vi "FPGA_CounterReadTimerOutput.vi"(8 "error in (no error)":errorcluster, 11 "Ctr Ref in":T1={"DevStatus"={"status"=FALSE, "code"=0, "source"=""}, "CntIndex"=enum."Ctr 1"}) -> (0 "error out":errorcluster, 1 "Stalled":bool, 2 "Period (s)":dbl, 3 "Ctr Ref out":T1={"DevStatus"={"status"=FALSE, "code"=0, "source"=""}, "CntIndex"=enum."Ctr 1"})   [LabVIEW 2017]
uses:
  <vilib>/Rock Robotics/SystemInterfaces/Counter/FPGA_CounterCtrDevRef.ctl
  <vilib>/Rock Robotics/SystemInterfaces/Counter/FPGA_CounterCtrSystemIndex.ctl
  <vilib>/Rock Robotics/SystemInterfaces/System/FPGA_SystemFPGA Ref Global.vi
  <vilib>/Utility/error.llb/Error Cluster From Error Code.vi
  <vilib>/rvi/errors/niLvFpgaAdjustHostInterfaceError.vi
  <vilib>/rvi/interface/nirviReadWriteControl/nirviReadWriteControl.xnode
  <vilib>/Rock Robotics/SystemInterfaces/System/FPGA_SystemFRC FPGA Ref.ctl
  NiFpgaLv.dll
  <vilib>/rvi/interface/Simulation/niFpgaSimulationCallBeginRW.vi
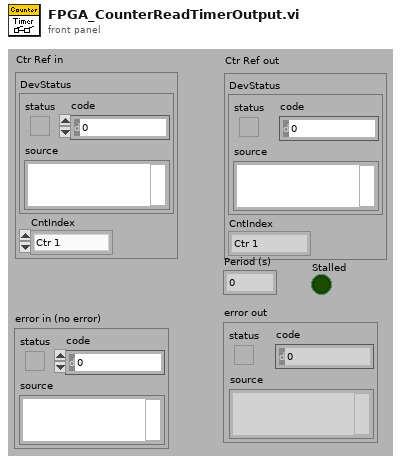
[diagram p1: front panel]
types:
  T1 = typedef "FPGA_CounterCtrDevRef.ctl" = cluster{"DevStatus":errorcluster, "CntIndex":T2}
  T2 = typedef "FPGA_CounterCtrSystemIndex.ctl" = enum8{"Ctr 0", "Ctr 1", "Ctr 2", "Ctr 3", "Ctr 4", "Ctr 5", "Ctr 6", "Ctr 7", "Invalid"}
  T3 = typedef "FPGA_SystemFRC FPGA Ref.ctl" = refnum<k20>
  T4 = cluster{"Period":fxp<+,23,24>, "Count":fxp<+/-,8,8>, "Stalled":bool}
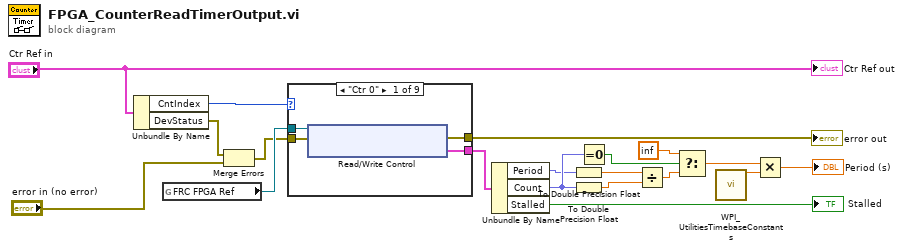
[diagram p0: block diagram]
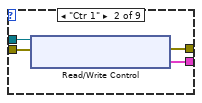
[diagram p2: hidden frame]
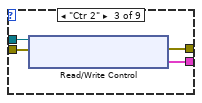
[diagram p3: hidden frame]
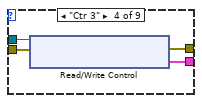
[diagram p4: hidden frame]
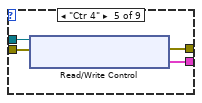
[diagram p5: hidden frame]
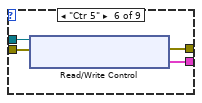
[diagram p6: hidden frame]
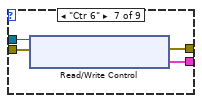
[diagram p7: hidden frame]
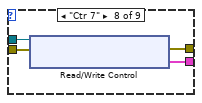
[diagram p8: hidden frame]
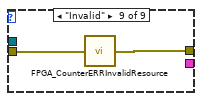
[diagram p9: hidden frame]
diagram:
  n1 = Unbundle By Name("Ctr Ref in") -> ("CntIndex"=w16:T2, "DevStatus"=w4:errorcluster)
  n2 = global read "FPGA_SystemFPGA Ref Global.vi" "FRC FPGA Ref"() -> (w6:T3)
  n3 = Merge Errors(w4, "error in (no error)") -> (w3:errorcluster)
  n4 = case shown="\"Ctr 0\"" w16 {
    tunnel: w6 -> [w22 w27 w31 w35 w39 w43 w47 w51 _]
    tunnel: w3 -> [w23 w26 w30 w34 w38 w42 w46 w50 w53]
    tunnel: [w21 w25 w29 w33 w37 w41 w45 w49 w52] -> w19
    tunnel: [w20 w24 w28 w32 w36 w40 w44 w48 _] -> w7
    frame "Ctr 0" {
      n5 = xnode "Read/Write Control"("FPGA VI Reference In"=w22, "error in"=w23) -> ("error out"=w21:errorcluster, "Counter0.TimerOutput"=w20:T4)  [unwired: 1 out]
    }
    frame "Ctr 1" {
      n6 = xnode "Read/Write Control"("FPGA VI Reference In"=w27, "error in"=w26) -> ("error out"=w25:errorcluster, "Counter1.TimerOutput"=w24:T4)  [unwired: 1 out]
    }
    frame "Ctr 2" {
      n7 = xnode "Read/Write Control"("FPGA VI Reference In"=w31, "error in"=w30) -> ("error out"=w29:errorcluster, "Counter2.TimerOutput"=w28:T4)  [unwired: 1 out]
    }
    frame "Ctr 3" {
      n8 = xnode "Read/Write Control"("FPGA VI Reference In"=w35, "error in"=w34) -> ("error out"=w33:errorcluster, "Counter3.TimerOutput"=w32:T4)  [unwired: 1 out]
    }
    frame "Ctr 4" {
      n9 = xnode "Read/Write Control"("FPGA VI Reference In"=w39, "error in"=w38) -> ("error out"=w37:errorcluster, "Counter4.TimerOutput"=w36:T4)  [unwired: 1 out]
    }
    frame "Ctr 5" {
      n10 = xnode "Read/Write Control"("FPGA VI Reference In"=w43, "error in"=w42) -> ("error out"=w41:errorcluster, "Counter5.TimerOutput"=w40:T4)  [unwired: 1 out]
    }
    frame "Ctr 6" {
      n11 = xnode "Read/Write Control"("FPGA VI Reference In"=w47, "error in"=w46) -> ("error out"=w45:errorcluster, "Counter6.TimerOutput"=w44:T4)  [unwired: 1 out]
    }
    frame "Ctr 7" {
      n12 = xnode "Read/Write Control"("FPGA VI Reference In"=w51, "error in"=w50) -> ("error out"=w49:errorcluster, "Counter7.TimerOutput"=w48:T4)  [unwired: 1 out]
    }
    frame "Invalid" {
      n13 = call <vilib>:"FPGA_CounterERRInvalidResource.vi"("error in (no error)"=w53) -> ("error out"=w52:errorcluster)
    }
  }
  "error out" <- w19
  n14 = Unbundle By Name(w7) -> ("Period"=w13:fxp<+,23,24>, "Count"=w14:fxp<+/-,8,8>, "Stalled"=→"Stalled":bool)
  n15 = To Double Precision Float(number=w13) -> (double precision float=w10:dbl)
  n16 = To Double Precision Float(number=w14) -> (double precision float=w12:dbl)
  n17 = Equal To 0?(x=w14) -> (x = 0?=w8:bool)
  n18 = Divide(x=w10, y=w12) -> (x/y=w11:dbl)
  n19 = Select(t=inf ("Period"), s=w8, f=w11) -> (s? t:f=w15:dbl)
  n20 = call <vilib>:"WPI_UtilitiesTimebaseConstants.vi"() -> ("40 MHz FPGA clock"=w2:dbl)  [unwired: 13 in, 2 out]
  n21 = Multiply(x=w15, y=w2) -> (x*y=→"Period (s)":dbl)
  "Ctr Ref out" <- "Ctr Ref in"
